vi "SlewRateLimiter_Example.vi"() -> ()   [LabVIEW 2019]
uses:
  <vilib>/Rock Robotics/WPI/ThirdParty/JAS_Junk/TrajLib/SlewRateLimiter_New.vi
  <vilib>/Rock Robotics/WPI/ThirdParty/JAS_Junk/TrajLib/SlewRateLimiter_Reset.vi
  <vilib>/Rock Robotics/WPI/ThirdParty/JAS_Junk/TrajLib/SlewRateLimiter_Calculate.vi
  <vilib>/Rock Robotics/WPI/ThirdParty/JAS_Junk/TrajLib/SlewRateLimiter_SetRate.vi
  <vilib>/Rock Robotics/WPI/ThirdParty/JAS_Junk/TrajLib/Util_GetTime.vi
  <vilib>/Rock Robotics/WPI/ThirdParty/JAS_Junk/TrajLib/Trajectory_Library.lvlib
panel:
  in  "Rate Limit  \nMax Units/Sec":dbl=10.0
  in  "Input":dbl(slide)=10.0 scale=-100.0..100.0 scale format="%12.2f"
  out "Rate Limited Output":dbl format="%12.2f"
  in  "Enable\nRate Lmiting":bool
  out "Trend":cluster{"Input":dbl, "Output":dbl}(graph)
  out "Rate Limiting \nEnabled":bool
  # "Slew Rate Limiter Sample"
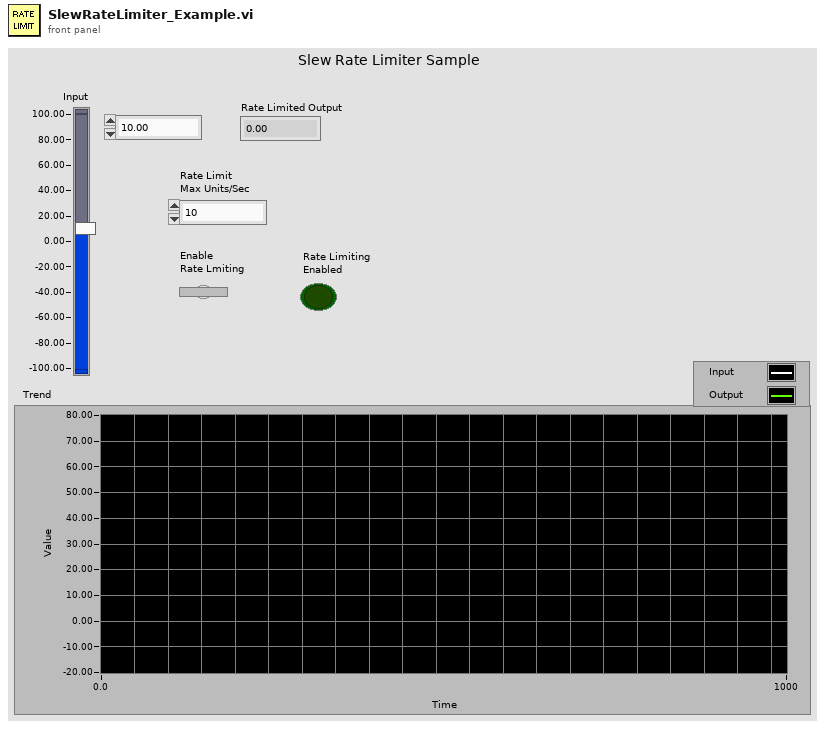
[diagram p1: front panel]
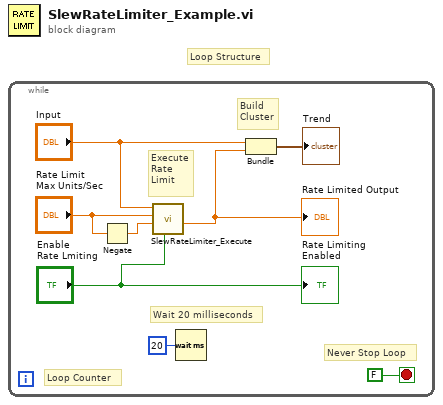
[diagram p0: block diagram]
diagram:
  # "Loop Structure"
  n1 = while {
    stop <- FALSE stop-if-true
    # "Execute\nRate\nLimit"
    # "Build\nCluster"
    # "Loop Counter"
    # "Never Stop Loop"
    # "Wait 20 milliseconds"
    n2 = Negate(x="Rate Limit  \nMax Units/Sec") -> (-x=w1:dbl)
    n3 = call <vilib>:"SlewRateLimiter_Execute.vi"("Enable"="Enable\nRate Lmiting", "NegativeRate"=w1, "PositiveRate"="Rate Limit  \nMax Units/Sec", "Input"="Input") -> ("Output"=w4:dbl)  [unwired: 6 in, 1 out]
    "Rate Limited Output" <- w4
    n4 = Wait (ms)(milliseconds to wait=u32 20) -> ()  [unwired: 1 out]
    n5 = Bundle("Input"="Input", "Output"=w4) -> (→"Trend":cluster{"Input":dbl, "Output":dbl})  [unwired: 1 in]
    "Rate Limiting \nEnabled" <- "Enable\nRate Lmiting"
  }
